vi "getMessage.vi"(8 "error in (no error)":errorcluster, 11 "TCPServer in":refnum<class "TCPServer.lvclass">) -> (0 "error out":errorcluster, 2 "String":string, 3 "TCPServer out":refnum<class "TCPServer.lvclass">)   [LabVIEW 2016, in "TCPServer.lvclass"]
uses:
  TCPServer.lvclass
  C:/Users/aanania/Desktop/TCPProtocol/TCPCommunicator/TCPCommunicator.lvclass
  TCPCommunicator/TCPCommunicator.lvclass/TCPCommunicator.ctl
  TCPComEvents/TCPComEvents.lvclass
  TCPSettings/TCPSettings.lvclass
  TCPCommunicator/TCPCommunicator.lvclass
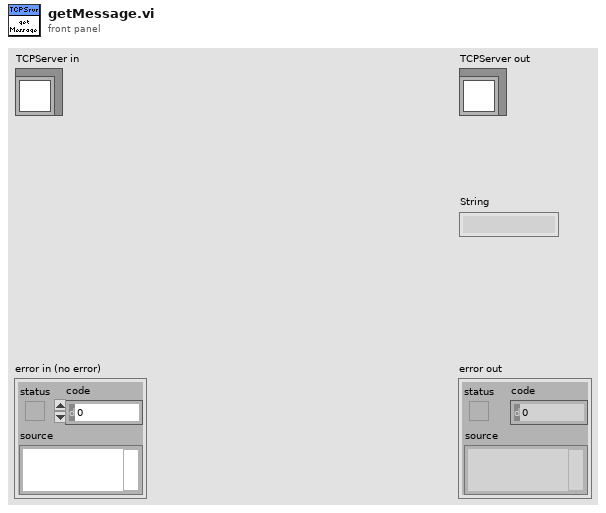
[diagram p1: front panel]
types:
  T1 = enum16{"Standard", "Buffered", "CRLF", "Immediate"}
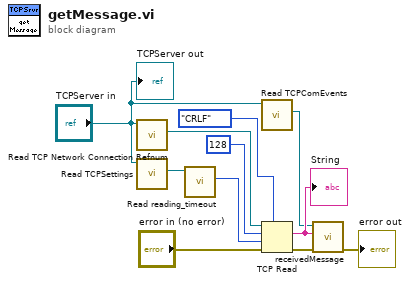
[diagram p0: block diagram]
diagram:
  n1 = call-dynamic "Read TCP Network Connection Refnum.vi"("TCPCommunicator in"="TCPServer in") -> ("TCP Network Connection Refnum"=w8:refnum<k5>)  [unwired: 8 in, 2 out]
  n2 = call-dynamic "Read TCPSettings.vi"("TCPCommunicator in"="TCPServer in") -> ("TCPSettings.lvclass"=w9:refnum<class "TCPSettings.lvclass">)  [unwired: 8 in, 2 out]
  n3 = call-dynamic "Read reading_timeout.vi"("TCPSettings in"=w9) -> ("reading_timeout"=w6:i32)  [unwired: 8 in, 2 out]
  n4 = call "Read TCPComEvents.vi"("TCPCommunicator in"="TCPServer in") -> ("TCPComEvents.lvclass"=w1:refnum<class "TCPComEvents.lvclass">)  [unwired: 8 in, 2 out]
  n5 = TCP Read(connection ID=w8, bytes to read=128, error in (no error)="error in (no error)", 7:T1."CRLF" ("mode (standard)"), 9:w6) -> (data out=w2:string, error out=w3:errorcluster)  [unwired: 1 out]
  "String" <- w2
  n6 = call "receivedMessage.vi"("error in (no error)"=w3, "message"=w2, "TCPComEvents in"=w1) -> ("error out"=→"error out":errorcluster)  [unwired: 7 in, 1 out]
  "TCPServer out" <- "TCPServer in"
